vi "Lim_FileOpenForRead.vi"(8 "error in (no error)":errorcluster, 10 "FilePath":path) -> (0 "error out":errorcluster, 3 "hFile":T1)   [LabVIEW 2014, in "ND2_Reader_32.lvlib"]
uses:
  ND2_Reader_32.lvlib
  controls/numeric_LIMFILEHANDLE.ctl
  nd2 reader/SDK/bin/x86/v6_w32_nd2ReadSDK.dll
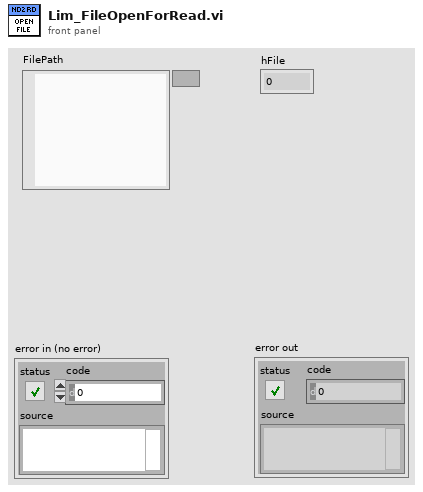
[diagram p1: front panel]
types:
  T1 = typedef "numeric_LIMFILEHANDLE.ctl" = i32
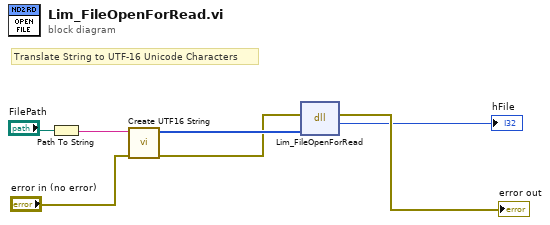
[diagram p0: block diagram]
diagram:
  # "Translate String to UTF-16 Unicode Characters"
  n1 = Path To String(path="FilePath") -> (string=w4:string)
  n2 = call "Create UTF16 String.vi"("error in (no error)"="error in (no error)", "ASCII string"=w4) -> ("error out"=w1:errorcluster, "UTF16 String"=w3:u16[])  [unwired: 4 in]
  n3 = dll-call lib="C:/Users/VirtualUser/Desktop/EPA-Vision/EPA Image Source LV2014 2.0.0 2016-02-23/ND2_Reader_32bit/nd2 reader/SDK/bin/x86/v6_w32_nd2ReadSDK.dll" fn="Lim_FileOpenForRead"(error in=w1, "wszFileName"=w3) -> (error out=→"error out":errorcluster, "LIMIFILEHANDLE"=→"hFile":i32)  [unwired: 2 in, 2 out]
